vi "2 NoSailGoodness.vi"(9 "Waypoint in":refnum<class "Waypoint.lvclass">, 10 "Heading to Test":dbl) -> (2 "Goodness":dbl)   [LabVIEW 2011]
doc: "Gives a goodness value to a test heading based on how it avoids no sail zones. All no sail zones of the current waypoint are considered. \n\nOutputs a value between 0 and 1 where 1 means the boat is not facing any no sail zones (they are more than 90 degrees away from the test heading) and 0 means the boat will go directly into a no sail zone if it maintains that test heading."
uses:
  2 Typedefs/UTM Circle.ctl
  2 Typedefs/UTM Location.ctl
  2 Classes/Waypoint/Waypoint.lvclass
  2 Globals/2 Global.vi
  2 Globals/2 TuningConstants.vi
panel:
  out "Robot UTM Location":T1 {"North" format="%#_10f"; "East" format="%#_8f"}
  out "No-sail circles considered":T2[](array[typedef])
  out "Tuning Quotient":dbl=0.05 step=0.1
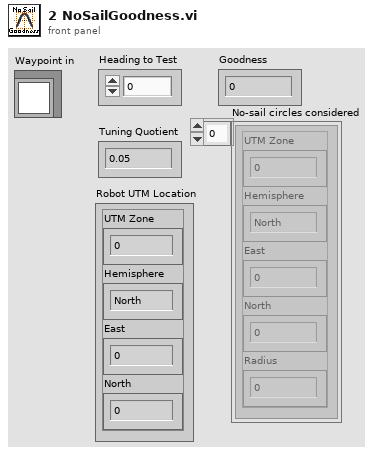
[diagram p1: front panel]
types:
  T1 = typedef "UTM Location.ctl" = cluster{"UTM Zone":dbl, "Hemisphere":enum16{"North", "South"}, "East":dbl, "North":dbl}
  T2 = typedef "UTM Circle.ctl" = cluster{"UTM Zone":dbl, "Hemisphere":enum16{"North", "South"}, "East":dbl, "North":dbl, "Radius":dbl}
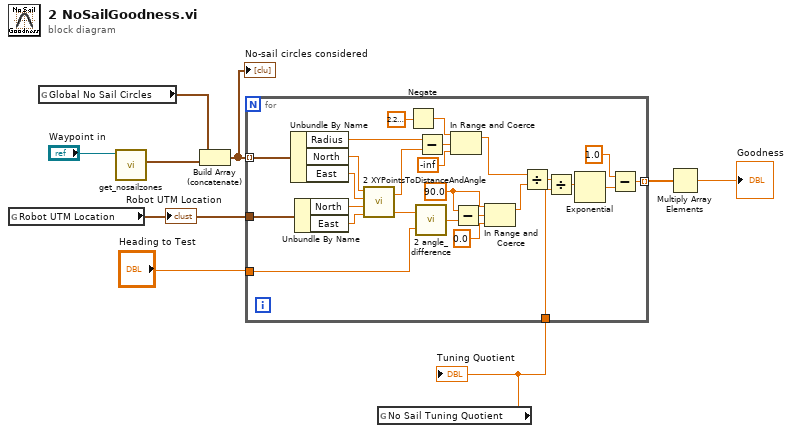
[diagram p0: block diagram]
diagram:
  n1 = global read "2 Global.vi" "Robot UTM Location"() -> (w8:T1)
  "Robot UTM Location" <- w8
  n2 = global read "2 Global.vi" "Global No Sail Circles"() -> (w5:T2[])
  n3 = call-dynamic "get_nosailzones.vi"("Waypoint in"="Waypoint in") -> ("No Sail Circles"=w4:T2[])  [unwired: 7 in, 2 out]
  n4 = Build Array (concatenate)(w5, w4) -> (w3:T2[])
  "No-sail circles considered" <- w3
  n5 = global read "2 TuningConstants.vi" "No Sail Tuning Quotient"() -> (w2:dbl)
  "Tuning Quotient" <- w2
  n6 = for {
    tunnel: "Heading to Test" -> [w28]
    tunnel: w3 -> [w35] mode=indexing
    tunnel: w8 -> [w34]
    tunnel: [w21] -> w7 mode=indexing
    tunnel: w2 -> [w10]
    w15 = 90.0
    n7 = Unbundle By Name(w35) -> ("Radius"=w27:dbl, "North"=w33:dbl, "East"=w32:dbl)
    n8 = Unbundle By Name(w34) -> ("North"=w31:dbl, "East"=w30:dbl)
    n9 = call "2 XYPointsToDistanceAndAngle.vi"("East 2"=w30, "North 2"=w31, "East 1"=w32, "North 1"=w33) -> ("Angle Diff"=w29:dbl, "Distance"=w26:dbl)
    n10 = Negate(x=2.220446049250313e-16) -> (-x=w13:dbl)
    n11 = call "2 angle_difference.vi"("Angle 2"=w28, "Angle 1"=w29) -> ("Difference"=w20:dbl)
    n12 = Subtract(x=w27, y=w26) -> (x-y=w25:dbl)
    n13 = In Range and Coerce(upper limit=w13, x=w25, lower limit=-inf) -> (coerced(x)=w24:dbl)  [unwired: 1 out]
    n14 = Subtract(x=w15, y=w20) -> (x-y=w19:dbl)
    n15 = In Range and Coerce(upper limit=w15, x=w19, lower limit=0.0) -> (coerced(x)=w17:dbl)  [unwired: 1 out]
    n16 = Divide(x=w24, y=w17) -> (x/y=w12:dbl)
    n17 = Divide(x=w12, y=w10) -> (x/y=w11:dbl)
    n18 = Exponential(1:w11) -> (0:w23:dbl)
    n19 = Subtract(x=1.0, y=w23) -> (x-y=w21:dbl)
  }
  n20 = Multiply Array Elements(1:w7) -> (0:→"Goodness":dbl)
